vi "test_UDP_Open connection using Clear Error node.vi"(8 "error in (no error)":errorcluster, 11 "TestCase in":refnum<class "Ethernet Protocol Tests.lvclass">) -> (0 "error out":errorcluster, 3 "TestCase out":refnum<class "Ethernet Protocol Tests.lvclass">)   [LabVIEW 2019, in "Ethernet Protocol Tests.lvclass"]
uses:
  Ethernet Protocol Tests.lvclass
  UDP/UDP.lvclass
  UDP/UDP.lvclass/UDP.ctl
  UDP/Data Access/Write Local IP Address.vi
  UDP/Data Access/Write Target IP Address.vi
  UDP/Data Access/Write Local Port.vi
  UDP/Data Access/Write Target Port.vi
  <vilib>/Utility/error.llb/Error Cluster From Error Code.vi
  <vilib>/ErrorRing/Error Ring.xnode
  <vilib>/addons/_JKI Toolkits/VI Tester/TestCase.llb/TestCase.lvclass
  C:/Program Files (x86)/National Instruments/LabVIEW 2019/vi.lib/addons/_JKI Toolkits/VI Tester/TestCase.llb/TestCase.lvclass
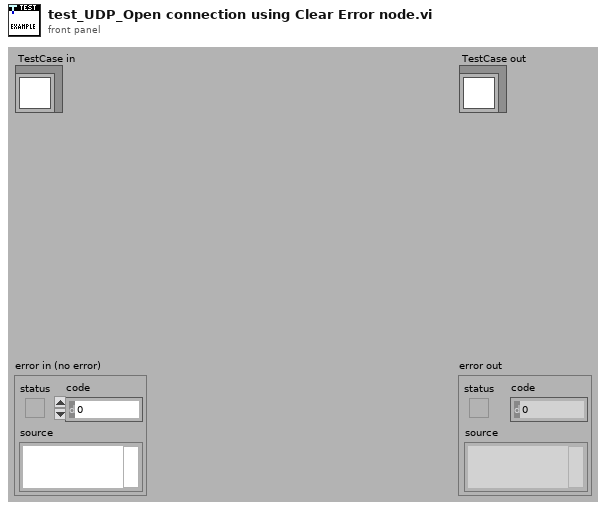
[diagram p1: front panel]
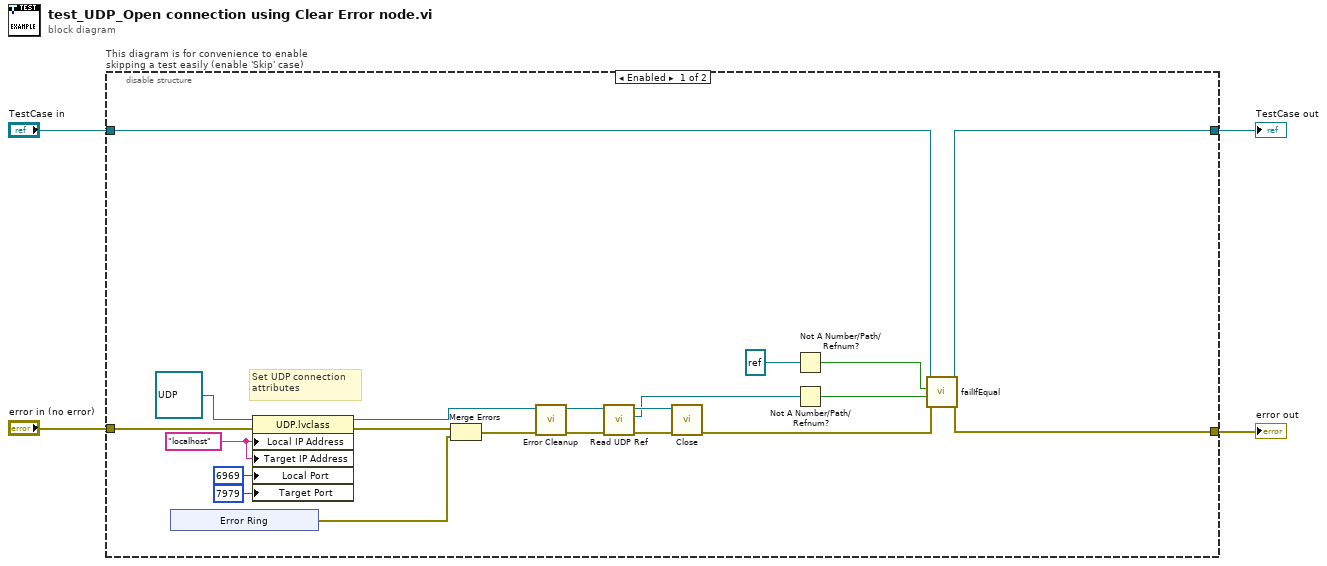
[diagram p0: block diagram]
diagram:
  n1 = disable-structure "This diagram is for convenience to enable skipping a test easily (enable 'Skip' case)" shown="Enabled" {
    disable-tunnel: "TestCase in" -> [w25 w34]
    disable-tunnel: [w24 w32] -> w1
    disable-tunnel: [w23 w33] -> w3
    disable-tunnel: "error in (no error)" -> [w21 w31]
    frame Enabled {
      w20 = "localhost" ("Local IP Address")
      # "Set UDP connection \nattributes"
      n2 = xnode "Error Ring"() -> ("error out"=w15:errorcluster)
      n3 = property class="UDP.lvclass"(reference=refnum<class "UDP.lvclass"> refnum ("Protocols.lvlib:UDP.lvclass"), error in=w21, "Local IP Address"=w20, "Target IP Address"=w20, "Local Port"=u16 6969, "Target Port"=u16 7979) -> (reference out=w14:refnum<class "UDP.lvclass">, error out=w17:errorcluster)
      n4 = Merge Errors(w17, w15) -> (w16:errorcluster)
      n5 = call-dynamic "Error Cleanup.vi"("error in (no error)"=w16, "UDP in"=w14) -> ("error out"=w12:errorcluster, "UDP out"=w11:refnum<class "UDP.lvclass">)  [unwired: 8 in]
      n6 = call "Read UDP Ref.vi"("error in (no error)"=w12, "UDP in"=w11) -> ("error out"=w10:errorcluster, "UDP Ref"=w8:refnum<k16>, "UDP out"=w9:refnum<class "UDP.lvclass">)  [unwired: 7 in]
      n7 = call-dynamic "Close.vi"("error in (no error)"=w10, "UDP in"=w9) -> ("error out"=w13:errorcluster)  [unwired: 8 in, 1 out]
      n8 = Not A Number/Path/Refnum?(number/path/refnum=refnum<k16> refnum ("UDP Ref")) -> (NaN/Path/Refnum?=w5:bool)
      n9 = Not A Number/Path/Refnum?(number/path/refnum=w8) -> (NaN/Path/Refnum?=w7:bool)
      n10 = call-dynamic "failIfEqual.vi"("error in (no error)"=w13, "y"=w7, "x"=w5, "TestCase in"=w25) -> ("error out"=w23:errorcluster, "TestCase out"=w24:refnum<class "Ethernet Protocol Tests.lvclass">)  [unwired: 6 in]
    }
    frame Disabled {
      # "skip test result while test is under development"
      n11 = call <vilib>:"skip.vi"("error in (no error)"=w31, "TestCase in"=w34) -> ("error out"=w33:errorcluster, "TestCase out"=w32:refnum<class "Ethernet Protocol Tests.lvclass">)  [unwired: 8 in]
    }
  }
  "error out" <- w3
  "TestCase out" <- w1
